vi "TestOpenFIle.vi"() -> ()   [LabVIEW 2018, in "ScratchpadLibrary.lvlib"]
uses:
  ScratchpadLibrary.lvlib
  <vilib>/platform/TimedLoop/XDataNode/XDataNode.xnode
  <vilib>/Platform/TimedLoop/XDataNode/nitl_modes.ctl
  <vilib>/Platform/TimedLoop/XDataNode/XDNodeRunTimeDep.lvlib
  <vilib>/Platform/TimedLoop/XDataNode/wakeup.ctl
  <vilib>/Platform/TimedLoop/XDataNode/timing_clust.ctl
panel:
  out "Log cycle":dbl
  out "Error":errorcluster
  out "File open error":errorcluster
  in  "File logging":bool caption="Start"
  out "Logging to file":bool
  out "File write error":errorcluster
  in  "Delimiter":string(combo)
  in  "Format":string(combo)
  out "Cycle":i32
  in  "stop":bool
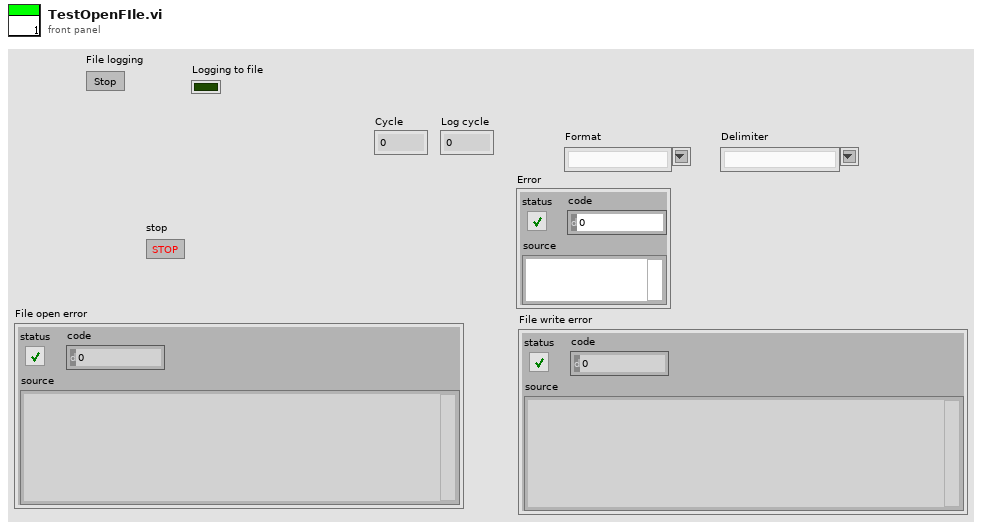
[diagram p1: front panel]
types:
  T1 = typedef "XDNodeRunTimeDep.lvlib/timing_clust.ctl" = cluster{"Expected End [f-1]":u64, "Actual End [f-1]":u64, "Finished Late? [f-1]":bool, "Expected End [i-1]":u64, "Actual End [i-1]":u64, "Finished Late? [i-1]":bool, "Expected Start [i]":u64, "Actual Start [i]":u64, "Expected Start [f]":u64, "Actual Start [f]":u64, "Source Name":string, "Structure Name":string, "Period":i64, "Deadline":i64, "Offset":i64, "Start":i64, "Priority":i32, "Timeout":i32, "Mode":T2, "Wakeup Reason":T3, "Error":errorcluster, "Source Type":string, "Secondary Source Type":string, "Global End Time":u64, "Global Start Time":u64, "Frame Duration":u64, "Iteration Duration":u64, "Assigned CPU":i32, "I/O Scan Engine Mode":u32}
  T2 = typedef "XDNodeRunTimeDep.lvlib/nitl_modes.ctl" = enum32{"No Change", "Process missed periods, maintain original phase", "Discard missed periods, maintain original phase", "Process missed periods, ignore original phase", "Discard missed periods, ignore original phase"}
  T3 = typedef "XDNodeRunTimeDep.lvlib/wakeup.ctl" = enum32{"Normal", "Aborted", "Asynchronous wakeup", "Timing source error", "Timed loop error", "Timeout"}
  T4 = enum16{"open", "replace", "create", "open or create", "replace or create", "replace or create with confirmation"}
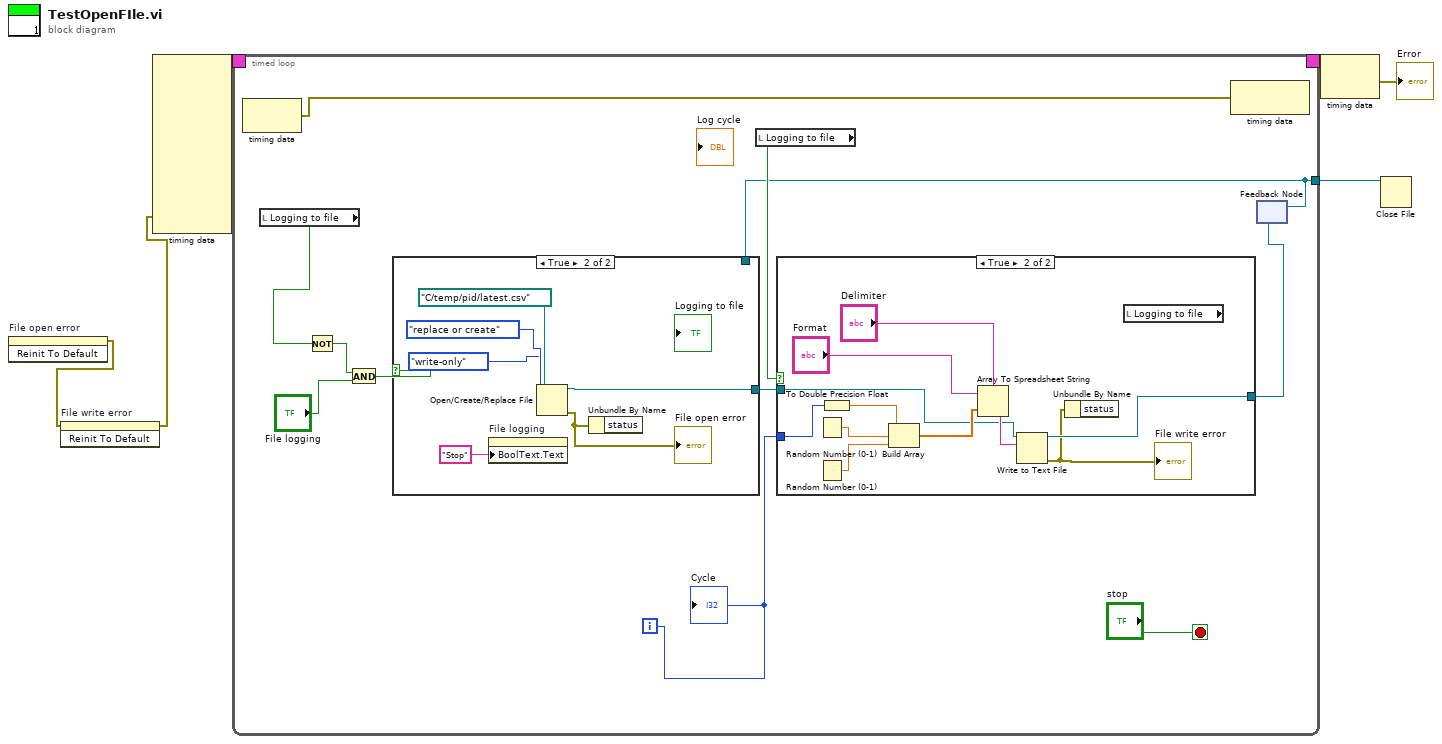
[diagram p0: block diagram]
diagram:
  n1 = invoke on="File open error" class="Clust (strict)" method="Reinit To Default"() -> (error out=w4:errorcluster)  [unwired: 3 in, 2 out]
  n2 = invoke on="File write error" class="Clust (strict)" method="Reinit To Default"(error in=w4) -> (error out=w3:errorcluster)  [unwired: 2 in, 2 out]
  n3 = node-c288(w3) -> (w6:T1)  [unwired: 9 in]
  n4 = timed-loop {
    timing: w6 -> [_]
    timing-out: [_] -> w5
    tunnel: [w7] -> w1
    i -> [w16]
    stop <- "stop" stop-if-true
    n5 = node-c288() -> (w9:errorcluster)  [unwired: 1 in]
    n6 = local read "Logging to file"() -> (w14:bool)
    n7 = Not(x=w14) -> (.not. x?=w12:bool)
    n8 = And(x=w12, y="File logging") -> (x .and. y?=w13:bool)
    n9 = local read "Logging to file"() -> (w15:bool)
    n10 = node-c288(w9) -> ()  [unwired: 1 out]
    n11 = feedback #1() -> (w7:refnum<file>)  [unwired: 1 in]
    n12 = case shown="True" w13 {
      tunnel: [w18 w23] -> w10
      tunnel: w7 -> [w18 _]
      frame False {
      }
      frame True {
        n13 = property on="File logging" class="Bool"("BoolText.Text"="Stop" ("Boolean Text.Text")) -> ()  [unwired: 2 in, 2 out]
        n14 = Open/Create/Replace File(file path (use dialog)=path "C:/temp/pid/latest.csv", operation (0:open)=T4."replace or create", access (0:read/write)=enum16{"read/write", "read-only", "write-only"}."write-only") -> (refnum out=w23:refnum<file>, cancelled=w24:bool, error out=w20:errorcluster)  [unwired: 3 in]
        "File open error" <- w20
        n15 = Unbundle By Name(w20) -> ("status"=w21:bool)
      }
    }
    n16 = case shown="True" w15 {
      tunnel: w16 -> [_ w42]
      tunnel: [w28 w34] -> w8
      tunnel: w10 -> [w28 w33]
      frame False {
      }
      frame True {
        n17 = Random Number (0-1)() -> (number: 0 to 1=w40:dbl)
        n18 = Random Number (0-1)() -> (number: 0 to 1=w39:dbl)
        n19 = To Double Precision Float(number=w42) -> (double precision float=w41:dbl)
        n20 = Build Array(w41, w40, w39) -> (w36:dbl[])
        n21 = Array To Spreadsheet String(delimiter (Tab)="Delimiter", array=w36, 3:"Format") -> (spreadsheet string=w35:string)
        n22 = Write to Text File(file (use dialog)=w33, text=w35) -> (refnum out=w34:refnum<file>, cancelled=w29:bool, error out=w31:errorcluster)  [unwired: 2 in]
        "File write error" <- w31
        n23 = Unbundle By Name(w31) -> ("status"=w30:bool)
        n24 = local read "Logging to file"() -> (w32:bool)
      }
    }
    n25 = feedback-in #1(w8) -> ()
    "Cycle" <- w16
  }
  n26 = node-c288(w5) -> (→"Error":errorcluster)
  n27 = Close File(refnum=w1) -> ()  [unwired: 1 in, 2 out]
